vi "Turn All Tubes ON-OFF.vi"(8 "Activate: 1\nDeactivate: 0":bool, 9 "Pins In":refnum<k21>[](array[refnum]), 10 "First Tube #":i32, 11 "Last Tube #":i32) -> (3 "Pins Out":refnum<k21>[](array[refnum]))   [LabVIEW 2020]
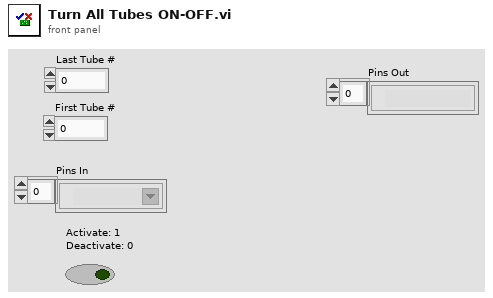
[diagram p1: front panel]
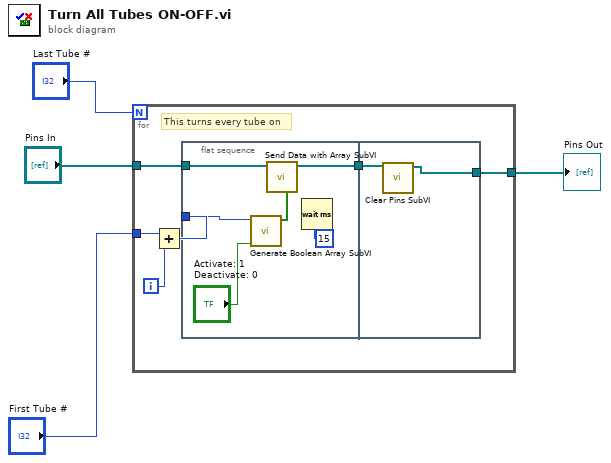
[diagram p0: block diagram]
diagram:
  n1 = for {
    N: "Last Tube #" -> [_]
    tunnel: "First Tube #" -> [w8]
    tunnel: "Pins In" -> [w7]
    tunnel: [w5] -> w2
    i -> [w9]
    # "This turns every tube on"
    n2 = Add(x=w8, y=w9) -> (x+y=w10:i32)
    n3 = flat-sequence {
      tunnel: [w15] -> w6
      tunnel: w7 -> [w12]
      tunnel: w10 -> [w13]
      tunnel: w6 -> [w18]
      tunnel: [w17] -> w5
      frame #0 {
        n4 = call "Generate Boolean Array SubVI.vi"("Activate: 1\nDeactivate: 0"="Activate: 1\nDeactivate: 0", "Tube"=w13) -> ("Boolean array"=w14:bool[])  [unwired: 9 in]
        n5 = call "Send Data with Array SubVI.vi"("Pins In"=w12, "Data"=w14) -> ("Pins Out"=w15:refnum<k21>[])  [unwired: 7 in]
        n6 = Wait (ms)(milliseconds to wait=u32 15) -> ()  [unwired: 1 out]
      }
      frame #1 {
        n7 = call "Clear Pins SubVI.vi"("Pins In"=w18) -> ("Pins Out"=w17:refnum<k21>[])  [unwired: 10 in]
      }
    }
  }
  "Pins Out" <- w2
